vi "Check for Regulation Target Crossing.vi"(6 "output power":dbl, 7 "first call?":bool, 8 "error in (no error)":errorcluster, 9 "previous measured value":dbl, 10 "results":T4, 11 "regulation settings":T1) -> (0 "error out":errorcluster, 1 "measured value":dbl, 3 "crossing found?":bool)   [LabVIEW 2021]
uses:
  controls/single tone audio measurements.ctl
  controls/regulation target.ctl
  controls/regulation target value units.ctl
  controls/audio controls.lvlib
  controls/regulation settings.ctl
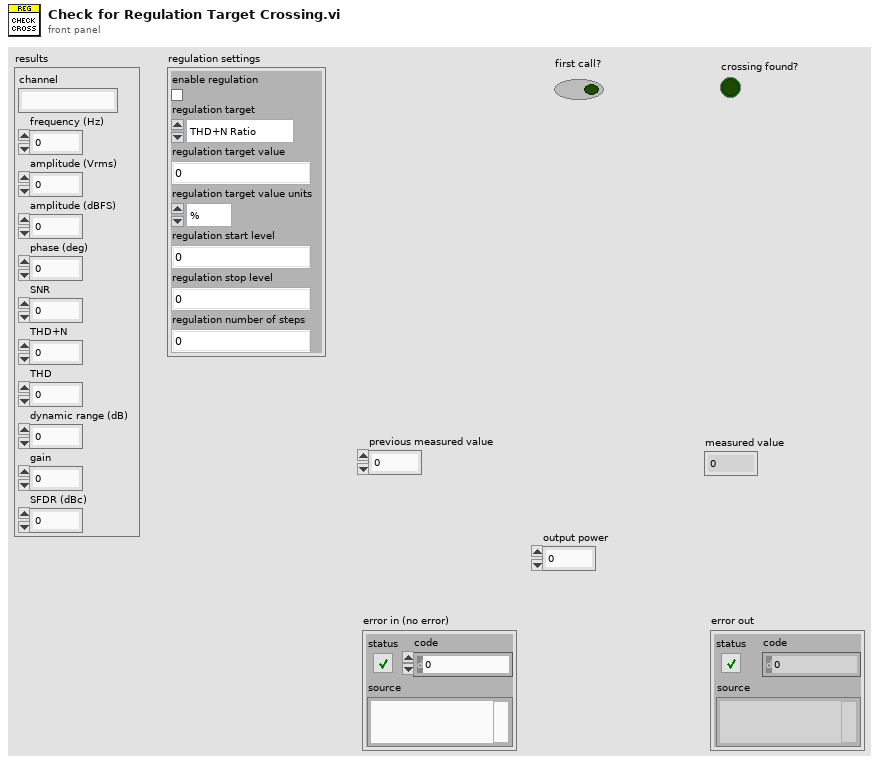
[diagram p1: front panel]
types:
  T1 = typedef "regulation settings.ctl" = cluster{"enable regulation":bool, "regulation target":T2, "regulation target value":dbl, "regulation target value units":T3, "regulation start level":dbl, "regulation stop level":dbl, "regulation number of steps":u32}
  T2 = typedef "regulation target.ctl" = enum32{"THD+N Ratio", "Output Power"}
  T3 = typedef "regulation target value units.ctl" = enum32{"%", "W"}
  T4 = typedef "audio controls.lvlib/single tone audio measurements.ctl" = cluster{"channel":string, "frequency (Hz)":dbl, "amplitude (Vrms)":dbl, "amplitude (dBFS)":dbl, "phase (deg)":dbl, "SNR":dbl, "THD+N":dbl, "THD":dbl, "dynamic range (dB)":dbl, "gain":dbl, "SFDR (dBc)":dbl}
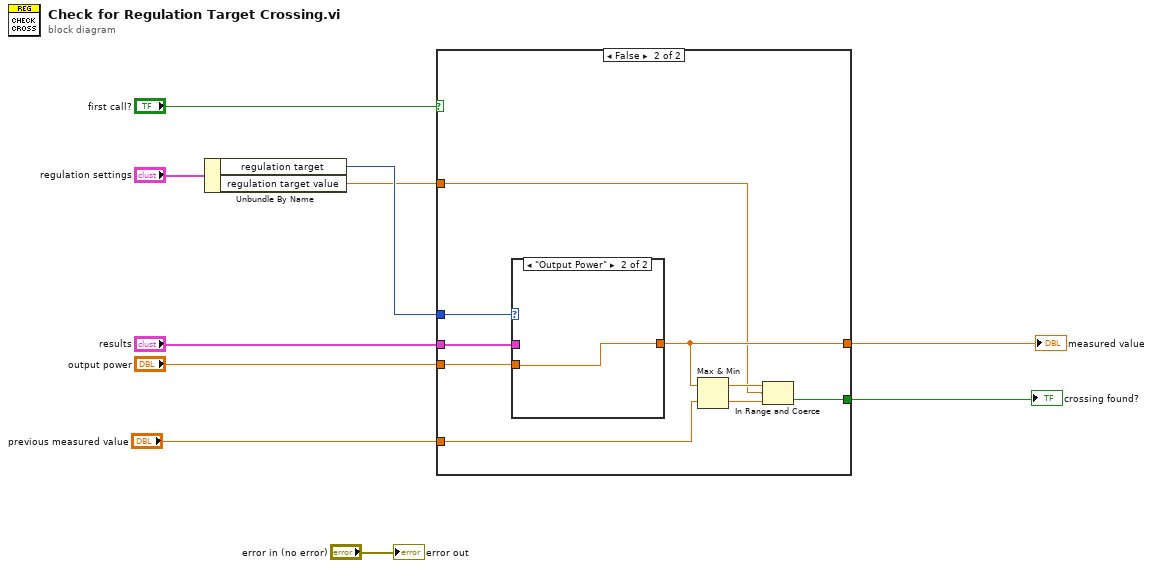
[diagram p0: block diagram]
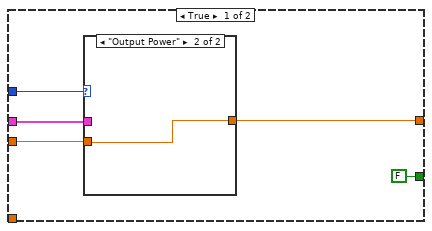
[diagram p2: hidden frame]
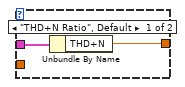
[diagram p3: hidden frame]
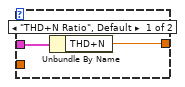
[diagram p4: hidden frame]
diagram:
  n1 = Unbundle By Name("regulation settings") -> ("regulation target"=w7:T2, "regulation target value"=w2:dbl)
  n2 = case shown="False" "first call?" {
    tunnel: "results" -> [w15 w27]
    tunnel: w7 -> [w14 w26]
    tunnel: "output power" -> [w13 w25]
    tunnel: [w12 w23] -> w5
    tunnel: "previous measured value" -> [_ w24]
    tunnel: w2 -> [_ w20]
    tunnel: [FALSE w19] -> w1
    frame True {
      n3 = case shown="\"Output Power\"" w14 {
        tunnel: w15 -> [w17 _]
        tunnel: [w16 w18] -> w12
        tunnel: w13 -> [_ w18]
        frame "THD+N Ratio", Default {
          n4 = Unbundle By Name(w17) -> ("THD+N"=w16:dbl)
        }
        frame "Output Power" {
        }
      }
    }
    frame False {
      n5 = case shown="\"Output Power\"" w26 {
        tunnel: w27 -> [w29 _]
        tunnel: [w28 w30] -> w23
        tunnel: w25 -> [_ w30]
        frame "THD+N Ratio", Default {
          n6 = Unbundle By Name(w29) -> ("THD+N"=w28:dbl)
        }
        frame "Output Power" {
        }
      }
      n7 = Max & Min(x=w23, y=w24) -> (max(x,y)=w22:dbl, min(x,y)=w21:dbl)
      n8 = In Range and Coerce(upper limit=w22, x=w20, lower limit=w21) -> (In Range?=w19:bool)  [unwired: 1 out]
    }
  }
  "crossing found?" <- w1
  "measured value" <- w5
  "error out" <- "error in (no error)"
